vi "niRFSysCalReader Initialize.vi"(8 "error in":errorcluster, 10 "Path Name":string, 11 "niRFSysCal XML File Path":path) -> (0 "error out":errorcluster, 3 "niRFSysCalReader Handle out":T1)   [LabVIEW 2018, in "niRFSysCalReader.lvlib"]
doc: "Creates a new niRFSysCalReader Handle."
uses:
  niRFSysCalReader.lvlib
  INCLUDES/niRFSysCalReader Handle.ctl
  INCLUDES/niRFSysCalReader CalPath Info.ctl
  INCLUDES/niRFSysCalReader Core States.ctl
  <vilib>/Utility/error.llb/Error Cluster From Error Code.vi
  <vilib>/ErrorRing/Error Ring.xnode
  Pathloss XML Reader/Pathloss XML Reader.lvlib
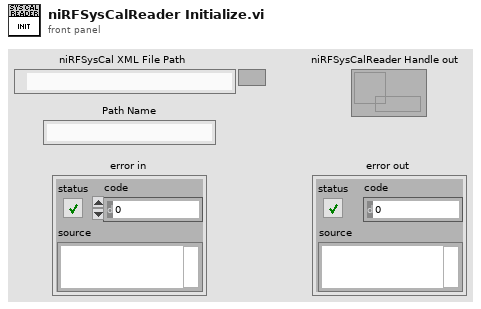
[diagram p1: front panel]
types:
  T1 = typedef "niRFSysCalReader.lvlib/niRFSysCalReader Handle.ctl" = refnum<data-value>
  T2 = typedef "niRFSysCalReader.lvlib/niRFSysCalReader CalPath Info.ctl" = cluster{"Path Name":string, "Path Type":string, "Path Source Port":string, "Path Destination Port":string, "Path Gain (dB)":dbl, "Cal Date":timestamp, "Cal Error Tolerance (dB)":dbl}
  T3 = typedef "niRFSysCalReader.lvlib/niRFSysCalReader Core States.ctl" = enum16{"Initialize", "Interpolator State", "Add CalData", "Get CalData", "Remove Pathloss", "Close"}
  T4 = typedef "Pathloss XML Reader.lvlib/XML Reader Data Ref.ctl" = refnum<data-value>
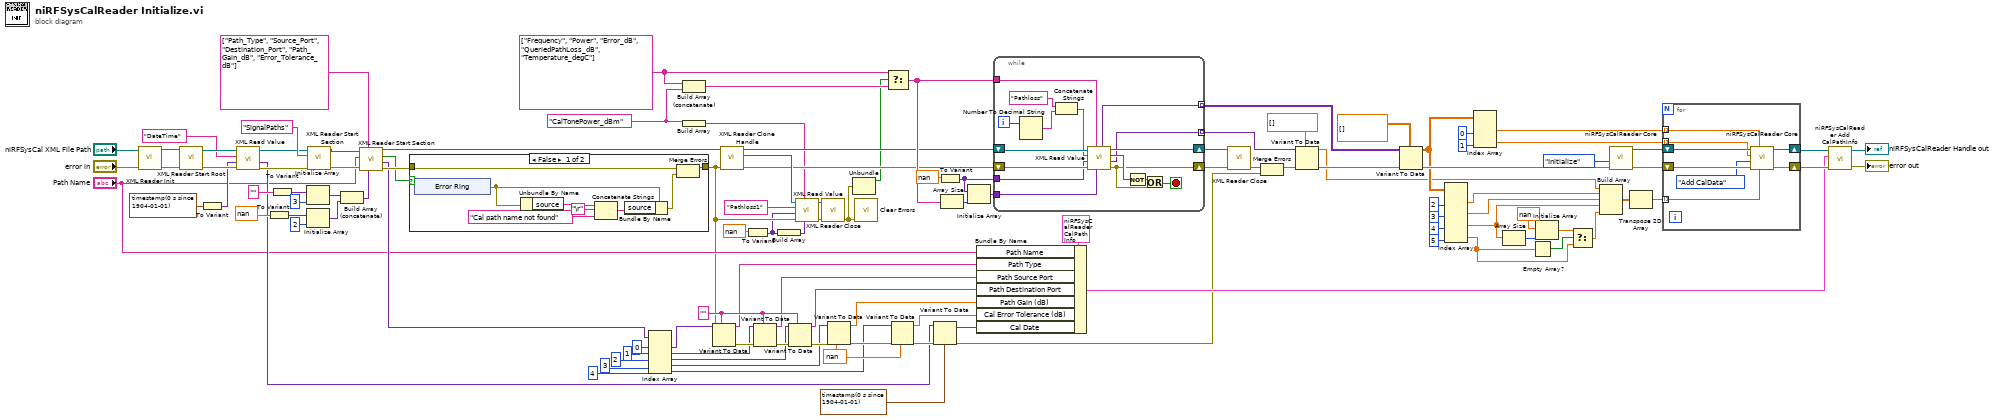
[diagram p0: block diagram]
diagram:
  w6 = "CalTonePower_dBm" ("Attribute Name")
  w47 = nan ("Default Element Value")
  w64 = ""
  w29 = string[] ["Frequency", "Power", "Error_dB", "QueriedPathLoss_dB", "Temperature_degC"] ("Attribute Names")
  n1 = call "XML Reader Init.vi"("error in"="error in", "File Path (dialog if empty)"="niRFSysCal XML File Path") -> ("error out"=w113:errorcluster, "XML Reader out"=w116:T4)  [unwired: 8 in]
  n2 = call "XML Reader Start Root.vi"("error in"=w113, "XML Reader In"=w116) -> ("error out"=w46:errorcluster, "XML Reader Out"=w45:T4)  [unwired: 8 in]
  n3 = To Variant(anything=timestamp(0 s since 1904-01-01) ("Cal Date")) -> (Variant=w40:variant)
  n4 = call "XML Read Value.vi"("error in (no error)"=w46, "Default Element Value"=w40, "Element Name"="DateTime", "XML Reader In"=w45) -> ("error out"=w42:errorcluster, "Element Value"=w38:variant, "XML Reader Out"=w43:T4)  [unwired: 3 in, 2 out]
  n5 = To Variant(anything=nan ("Default Element Value")) -> (Variant=w76:variant)
  n6 = To Variant(anything="") -> (Variant=w77:variant)
  n7 = Initialize Array(w77, 3 ("dimension size")) -> (w78:variant[])
  n8 = Initialize Array(w76, 2 ("dimension size")) -> (w74:variant[])
  n9 = call "XML Reader Start Section.vi"("error in"=w42, "Element Name"="SignalPaths" ("Section Name"), "XML Reader In"=w43) -> ("error out"=w112:errorcluster, "XML Reader Out"=w111:T4)  [unwired: 5 in, 2 out]
  n10 = Build Array (concatenate)(w78, w74) -> (w79:variant[])
  n11 = call "XML Reader Start Section.vi"("Default Attribute Values"=w79, "Attribute Names"=string[] ["Path_Type", "Source_Port", "Destination_Port", "Path_Gain_dB", "Error_Tolerance_dB"], "error in"=w112, "Element Name"="Path Name", "XML Reader In"=w111) -> ("error out"=w110:errorcluster, "Attribute Values"=w72:variant[], "Found?"=w93:bool, "XML Reader Out"=w13:T4)  [unwired: 3 in]
  n12 = case shown="False" w93 {
    tunnel: w110 -> [w123 w129]
    tunnel: [w124 w129] -> w10
    frame False {
      n13 = xnode "Error Ring"() -> ("error out"=w122:errorcluster)
      n14 = Unbundle By Name(w122) -> ("source"=w119:string)
      n15 = Concatenate Strings(w119, "\r", "Cal path name not found" ("error message (\"\")")) -> (w120:string)
      n16 = Bundle By Name(cluster=w122, "source"=w120) -> (w121:errorcluster)
      n17 = Merge Errors(w123, w121) -> (w124:errorcluster)
    }
    frame True {
    }
  }
  n18 = Index Array(array=w72, index #1=0 ("index"), index #2=1 ("index"), index #3=2 ("index"), index #4=3 ("index"), index #5=4 ("index")) -> (element #1=w62:variant, element #2=w56:variant, element #3=w55:variant, element #4=w53:variant, element #5=w32:variant)
  n19 = Build Array (concatenate)(w29, w6) -> (w28:string[])
  n20 = Build Array(w6) -> (w5:string[])
  n21 = Variant To Data(error in=w10, type=w64, Variant=w62) -> (data=w18:string, error out=w66:errorcluster)
  n22 = call "XML Reader Clone Handle.vi"("error in (no error)"=w10, "XML Reader In"=w13) -> ("error out"=w9:errorcluster, "XML Reader Copy"=w11:refnum<data-value>, "XML Reader Out"=w12:T4)  [unwired: 7 in]
  n23 = To Variant(anything=nan ("Default Element Value")) -> (Variant=w8:variant)
  n24 = Variant To Data(error in=w66, type=w64, Variant=w56) -> (data=w51:string, error out=w65:errorcluster)
  n25 = Build Array(w8) -> (w7:variant[])
  n26 = Variant To Data(error in=w65, type=w64, Variant=w55) -> (data=w50:string, error out=w54:errorcluster)
  n27 = call "XML Read Value.vi"("Default Attribute Values"=w7, "Attribute Names"=w5, "error in (no error)"=w10, "Default Element Value"=w8, "Element Name"="Pathloss1" ("string"), "XML Reader In"=w11) -> ("error out"=w3:errorcluster, "XML Reader Out"=w4:T4)  [unwired: 1 in, 3 out]
  n28 = call "XML Reader Close.vi"("error in"=w3, "XML Reader In"=w4) -> ("error out"=w2:errorcluster)  [unwired: 9 in]
  n29 = Variant To Data(error in=w54, type=w47, Variant=w53) -> (data=w49:dbl, error out=w52:errorcluster)
  n30 = Unbundle(w2) -> ("status"=w1:bool)  [unwired: 2 out]
  n31 = call <vilib>:"Clear Errors.vi"("error in (no error)"=w2) -> ()  [unwired: 5 in, 2 out]
  n32 = Select(t=w29, s=w1, f=w28) -> (s? t:f=w16:string[])
  n33 = Variant To Data(error in=w52, type=w47, Variant=w32) -> (data=w48:dbl, error out=w39:errorcluster)
  n34 = Variant To Data(error in=w39, type=timestamp(0 s since 1904-01-01) ("Cal Date"), Variant=w38) -> (data=w36:timestamp, error out=w34:errorcluster)
  n35 = To Variant(anything=nan ("Default Element Value")) -> (Variant=w101:variant)
  n36 = Array Size(array=w16) -> (size(s)=w17:i32)
  n37 = Initialize Array(w101, w17) -> (w102:variant[])
  n38 = Bundle By Name(cluster=T2 {"Path Name"="", "Path Type"="", "Path Source Port"="", "Path Destination Port"="", "Path Gain (dB)"=0.0, "Cal Date"=timestamp(0 s since 1904-01-01), "Cal Error Tolerance (dB)"=0.0} ("CalPath Info"), "Path Name"="Path Name", "Path Type"=w18, "Path Source Port"=w51, "Path Destination Port"=w50, "Path Gain (dB)"=w49, "Cal Error Tolerance (dB)"=w48, "Cal Date"=w36) -> (w63:T2)
  n39 = while {
    tunnel: w101 -> [w138]
    tunnel: [w134] -> w108 mode=indexing
    tunnel: w16 -> [w132]
    tunnel: w102 -> [w131]
    tunnel: [w130] -> w105 mode=indexing
    shift-right: [w136] -> w107
    shift-left: w9 -> [w144]
    shift-right: [w143] -> w109
    shift-left: w12 -> [w145]
    i -> [w142]
    stop <- w135 stop-if-true
    n40 = Number To Decimal String(number=w142) -> (decimal integer string=w140:string)  [unwired: 1 in]
    n41 = Concatenate Strings("Pathloss" ("string"), w140) -> (w139:string)
    n42 = call "XML Read Value.vi"("Default Attribute Values"=w131, "Attribute Names"=w132, "error in (no error)"=w144, "Default Element Value"=w138, "Element Name"=w139, "XML Reader In"=w145) -> ("error out"=w136:errorcluster, "Element Value"=w134:variant, "Found?"=w137:bool, "XML Reader Out"=w143:T4, "Attribute Values"=w130:variant[])  [unwired: 1 in]
    n43 = Not(x=w137) -> (.not. x?=w133:bool)
    n44 = Or(x=w133, y=w136) -> (x .or. y?=w135:bool)
  }
  n45 = call "XML Reader Close.vi"("error in"=w107, "XML Reader In"=w109) -> ("error out"=w106:errorcluster)  [unwired: 9 in]
  n46 = Merge Errors(w106, w34) -> (w35:errorcluster)
  n47 = Variant To Data(error in=w35, type=dbl[] [], Variant=w108) -> (data=w20:dbl[], error out=w104:errorcluster)
  n48 = Variant To Data(error in=w104, type=dbl[][] [], Variant=w105) -> (data=w92:dbl[][], error out=w99:errorcluster)
  n49 = Index Array(array=w92, index (col) #1=2 ("disabled index (col)"), index (col) #2=3 ("index (col)"), index (col) #3=4 ("index (col)"), index (col) #4=5 ("index (col)")) -> (element #1=w87:dbl[], element #2=w86:dbl[], element #3=w25:dbl[], element #4=w19:dbl[])  [unwired: 4 in]
  n50 = Index Array(array=w92, index (col) #1=0 ("disabled index (col)"), index (col) #2=1 ("index (col)")) -> (element #1=w96:dbl[], element #2=w85:dbl[])  [unwired: 2 in]
  n51 = Array Size(array=w25) -> (size(s)=w24:i32)
  n52 = Empty Array?(array=w19) -> (empty?=w26:bool)
  n53 = Initialize Array(nan ("element"), w24) -> (w22:dbl[])
  n54 = Select(t=w22, s=w26, f=w19) -> (s? t:f=w21:dbl[])
  n55 = Build Array(w20, w87, w86, w25, w21) -> (w84:dbl[][])
  n56 = call "niRFSysCalReader Core.vi"("error in"=w99, "niRFSysCalReader State"=niRFSysCalReader_Core_States."Initialize" ("Cal Storage")) -> ("error out"=w98:errorcluster, "niRFSysCalReader Handle out"=w95:T1)  [unwired: 7 in, 1 out]
  n57 = Transpose 2D Array(2D array=w84) -> (transposed array=w83:dbl[][])
  n58 = for {
    shift-right: [w153] -> w68
    shift-left: w98 -> [w152]
    tunnel: w96 -> [w149] mode=indexing
    shift-right: [w150] -> w71
    shift-left: w95 -> [w151]
    tunnel: w85 -> [w148] mode=indexing
    tunnel: w83 -> [w147] mode=indexing
    n59 = call "niRFSysCalReader Core.vi"("CalData"=w147, "Frequency (Hz)"=w149, "error in"=w152, "niRFSysCalReader State"=niRFSysCalReader_Core_States."Add CalData", "Power (dBm)"=w148, "niRFSysCalReader Handle"=w151) -> ("error out"=w153:errorcluster, "niRFSysCalReader Handle out"=w150:T1)  [unwired: 3 in, 1 out]
  }
  n60 = call "niRFSysCalReader Add CalPathInfo.vi"("error in"=w68, "CalPath Info"=w63, "niRFSysCalReader Handle"=w71) -> ("error out"=→"error out":errorcluster, "niRFSysCalReader Handle out"=→"niRFSysCalReader Handle out":T1)  [unwired: 7 in]
